vi "SmartSEM Remote API initialization status.vi"(8 "error in":errorcluster, 11 "ActiveX Container":refnum<k7>(container)) -> (0 "error out":errorcluster, 1 "API initialized":bool, 3 "reference out":refnum<k7>)   [LabVIEW 2018]
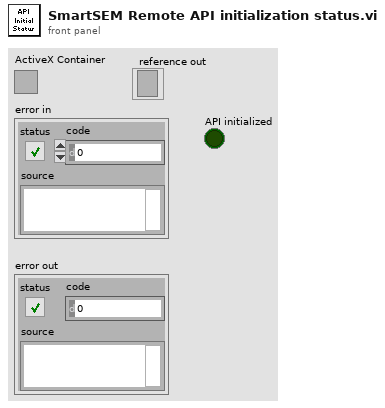
[diagram p1: front panel]
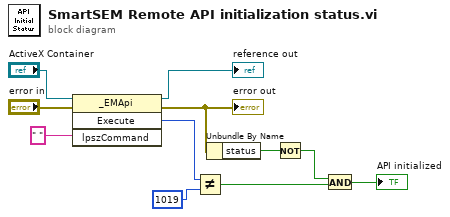
[diagram p0: block diagram]
diagram:
  n1 = invoke class="_EMApi" method="Execute"(reference="ActiveX Container", error in="error in", "lpszCommand"=" " ("lpszUserName")) -> (reference out=→"reference out":refnum<k7>, error out=w7:errorcluster, "Execute"=w10:i32)  [unwired: 1 in, 1 out]
  "error out" <- w7
  n2 = Not Equal?(x=w10, y=1019) -> (x != y?=w3:bool)
  n3 = Unbundle By Name(w7) -> ("status"=w6:bool)
  n4 = Not(x=w6) -> (.not. x?=w4:bool)
  n5 = And(x=w4, y=w3) -> (x .and. y?=→"API initialized":bool)
